vi "Eraze_Cal_vals.vi"(8 "error in (no error)":errorcluster, 10 "Eraze":bool, 11 "USB Interface Name":refnum<visa-resource-name>="COM3") -> (0 "error out":errorcluster, 3 "String":string)   [LabVIEW 2012]
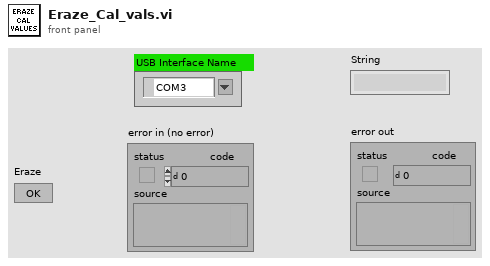
[diagram p1: front panel]
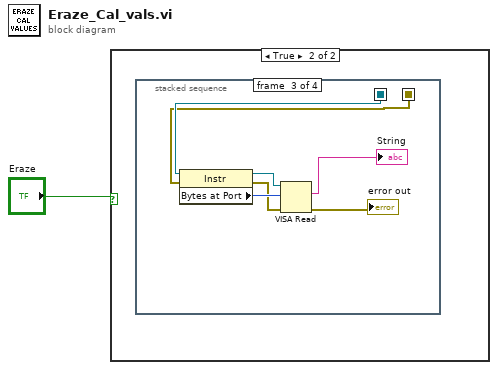
[diagram p0: block diagram]
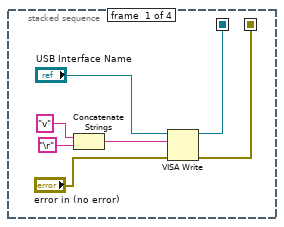
[diagram p3: hidden frame]
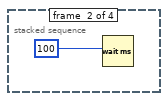
[diagram p4: hidden frame]
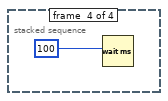
[diagram p5: hidden frame]
diagram:
  n1 = case shown="True" "Eraze" {
    frame False {
    }
    frame True {
      n2 = stacked-sequence {
        seq-local: [w4 _ _ _] -> [_ _ w14 _]
        seq-local: [w2 _ _ _] -> [_ _ w13 _]
        frame #0 {
          n3 = Concatenate Strings("v", "\r") -> (w6:string)
          n4 = VISA Write(VISA resource name="USB Interface Name", write buffer=w6, error in (no error)="error in (no error)") -> (VISA resource name out=w4:refnum<visa-resource-name>, error out=w2:errorcluster)  [unwired: 1 out]
        }
        frame #1 {
          n5 = Wait (ms)(milliseconds to wait=100) -> ()  [unwired: 1 out]
        }
        frame #2 {
          n6 = property class="Instr"(reference=w14, error in=w13) -> (reference out=w11:refnum<visa-resource-name>, error out=w12:errorcluster, "Bytes at Port"=w15:u32)
          n7 = VISA Read(VISA resource name=w11, byte count=w15, error in (no error)=w12) -> (read buffer=→"String":string, error out=→"error out":errorcluster)  [unwired: 2 out]
        }
        frame #3 {
          n8 = Wait (ms)(milliseconds to wait=100) -> ()  [unwired: 1 out]
        }
      }
    }
  }
